vi "Release Target Timing Source.vi"(8 "error in (no error)":errorcluster, 11 "CD Ref in":T1 format="%.0x") -> (0 "error out":errorcluster, 3 "CD Ref out":T1 format="%.0x")   [LabVIEW 2019, in "TimingDRV System Explorer.lvlib"]
uses:
  TimingDRV System Explorer.lvlib
  <vilib>/NI VeriStand/Custom Device API/Custom Device Item Ref.ctl
  NationalInstruments.VeriStand.SystemDefinitionAPI
  NationalInstruments.VeriStand.SystemStorage
  <vilib>/NI VeriStand/Custom Device Tools/Custom Device Utility Library/Custom Device Utility Library.lvlib
  <vilib>/NI VeriStand/Custom Device API/Custom Device API.lvlib
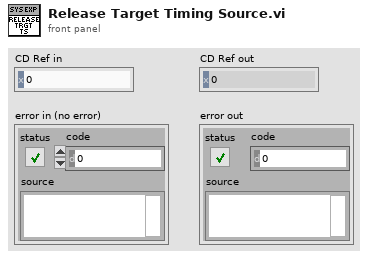
[diagram p1: front panel]
types:
  T1 = typedef "Custom Device API.lvlib/Custom Device Item Ref.ctl" = u64
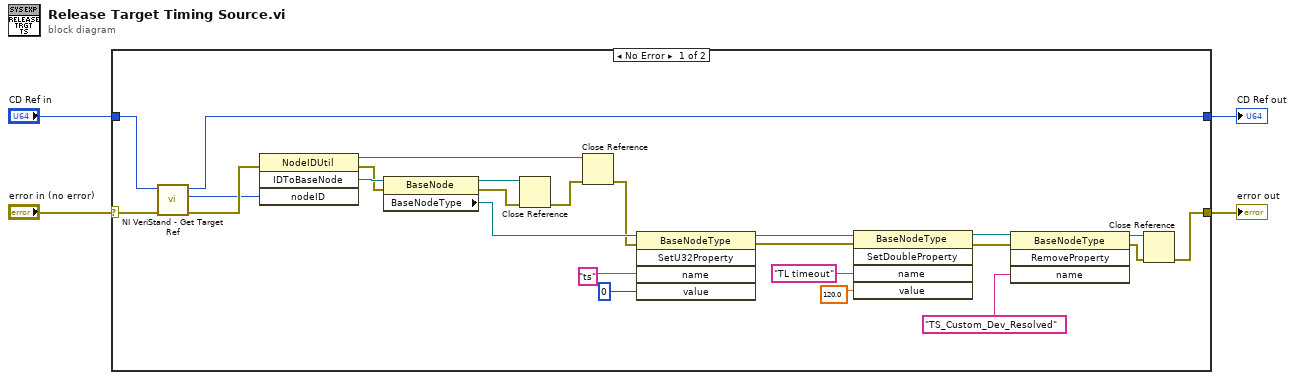
[diagram p0: block diagram]
diagram:
  n1 = case shown="No Error" "error in (no error)" {
    selector: "error in (no error)" -> [w27 w30]
    tunnel: [w7 w30] -> w4
    tunnel: [w29 w31] -> w3
    tunnel: "CD Ref in" -> [w28 w31]
    frame No Error {
      n2 = call <vilib>:"NI VeriStand - Get Target Ref.vi"("error in"=w27, "Item Ref in"=w28) -> ("error out"=w9:errorcluster, "Target Ref"=w8:T1, "Item Ref out"=w29:T1)  [unwired: 6 in, 1 out]
      n3 = invoke class="NodeIDUtil" method="IDToBaseNode"(error in=w9, "nodeID"=w8) -> (reference out=w22:refnum<k24>, error out=w23:errorcluster, "IDToBaseNode"=w24:refnum<k24>)  [unwired: 2 in, 1 out]
      n4 = property class="BaseNode"(reference=w24, error in=w23) -> (reference out=w20:refnum<k24>, error out=w21:errorcluster, "BaseNodeType"=w26:refnum<k24>)
      n5 = Close Reference(reference=w20, error in (no error)=w21) -> (error out=w19:errorcluster)
      n6 = Close Reference(reference=w22, error in (no error)=w19) -> (error out=w25:errorcluster)
      n7 = invoke class="BaseNodeType" method="SetU32Property"(reference=w26, error in=w25, "name"="ts", "value"=u32 0) -> (reference out=w15:refnum<k24>, error out=w18:errorcluster)  [unwired: 1 in, 3 out]
      n8 = invoke class="BaseNodeType" method="SetDoubleProperty"(reference=w15, error in=w18, "name"="TL timeout", "value"=120.0) -> (reference out=w16:refnum<k24>, error out=w17:errorcluster)  [unwired: 1 in, 3 out]
      n9 = invoke class="BaseNodeType" method="RemoveProperty"(reference=w16, error in=w17, "name"="TS_Custom_Dev_Resolved") -> (reference out=w5:refnum<k24>, error out=w6:errorcluster)  [unwired: 1 in, 2 out]
      n10 = Close Reference(reference=w5, error in (no error)=w6) -> (error out=w7:errorcluster)
    }
    frame Error {
    }
  }
  "error out" <- w4
  "CD Ref out" <- w3
